vi "_Linear Interpolation.vi"(0 "X1":dbl, 1 "X2":dbl, 2 "Y1":dbl, 3 "Y2":dbl, 4 "X":dbl) -> (5 "Y":dbl, 6 "Slope":dbl)   [LabVIEW 2015]
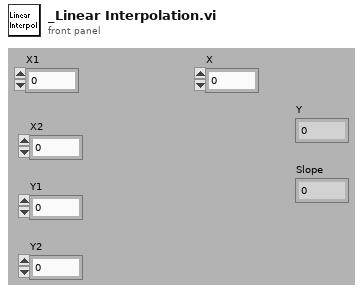
[diagram p1: front panel]
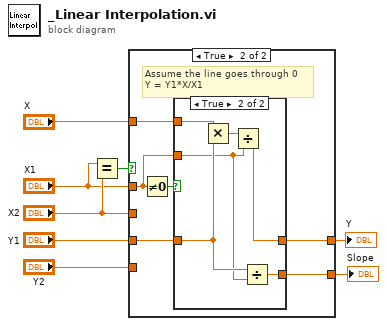
[diagram p0: block diagram]
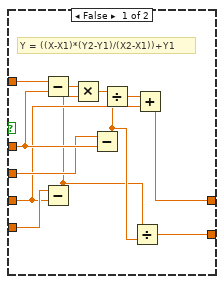
[diagram p2: hidden frame]
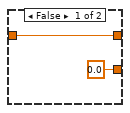
[diagram p3: hidden frame]
diagram:
  n1 = Equal?(x="X1", y="X2") -> (x = y?=w6:bool)
  n2 = case shown="True" w6 {
    tunnel: "X1" -> [w17 w23]
    tunnel: "X2" -> [w16 _]
    tunnel: "Y1" -> [w13 w25]
    tunnel: "Y2" -> [w18 _]
    tunnel: [w12 w24] -> w4
    tunnel: "X" -> [w20 w22]
    tunnel: [w9 w21] -> w1
    frame False {
      # "Y = ((X-X1)*(Y2-Y1)/(X2-X1))+Y1"
      n3 = Subtract(x=w20, y=w17) -> (x-y=w19:dbl)
      n4 = Subtract(x=w18, y=w13) -> (x-y=w10:dbl)
      n5 = Multiply(x=w19, y=w10) -> (x*y=w15:dbl)
      n6 = Subtract(x=w16, y=w17) -> (x-y=w11:dbl)
      n7 = Divide(x=w15, y=w11) -> (x/y=w14:dbl)
      n8 = Divide(x=w10, y=w11) -> (x/y=w9:dbl)
      n9 = Add(x=w14, y=w13) -> (x+y=w12:dbl)
    }
    frame True {
      # "Assume the line goes through 0\nY = Y1*X/X1"
      n10 = Not Equal To 0?(x=w23) -> (x != 0?=w26:bool)
      n11 = case shown="True" w26 {
        tunnel: [w28 w32] -> w24
        tunnel: w25 -> [w28 w31]
        tunnel: w23 -> [_ w30]
        tunnel: w22 -> [_ w34]
        tunnel: [0.0 w29] -> w21
        frame False {
        }
        frame True {
          n12 = Multiply(x=w34, y=w31) -> (x*y=w33:dbl)
          n13 = Divide(x=w33, y=w30) -> (x/y=w32:dbl)
          n14 = Divide(x=w31, y=w30) -> (x/y=w29:dbl)
        }
      }
    }
  }
  "Y" <- w4
  "Slope" <- w1
